vi "Counter with Load and Rollover_2016.vi"(8 "INC?":bool, 9 "Load Value":u64, 10 "Load?":bool) -> (3 "count":u64)   [LabVIEW 2016]
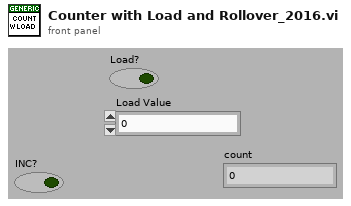
[diagram p1: front panel]
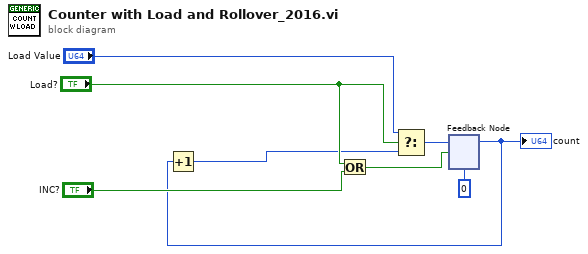
[diagram p0: block diagram]
diagram:
  n1 = Or(x="Load?", y="INC?") -> (x .or. y?=w3:bool)
  n2 = feedback #1(u64 0) -> (w2:u64)
  "count" <- w2
  n3 = Increment(x=w2) -> (x+1=w1:u64)
  n4 = Select(t="Load Value", s="Load?", f=w1) -> (s? t:f=w4:u64)
  n5 = feedback-in #1(w4, w3) -> ()
